vi "Global Log Event Example.vi"() -> ()   [LabVIEW 2017]
uses:
  user.lib/_NEVSTOP/Communicable State Machine(CSM)/_Support/Typedef/_CSM_GlobalLog_MSG.ctl
  user.lib/_NEVSTOP/Communicable State Machine(CSM)/_Support/Typedef/_CSM_Response Source Message.ctl
  user.lib/_NEVSTOP/Communicable State Machine(CSM)/_Support/Typedef/_CSM_GlobalLog_MSG_TYPE.ctl
  user.lib/_NEVSTOP/Communicable State Machine(CSM)/AdvanceAPI/CSM - Convert Error to Argument.vi
  user.lib/_NEVSTOP/Communicable State Machine(CSM)/_Support/GlobalEvent/GEvt-Generate with Rule Check.vi
  user.lib/_NEVSTOP/Communicable State Machine(CSM)/_Support/GlobalEvent/Cache-GEvt Refs.vi
  user.lib/_NEVSTOP/Communicable State Machine(CSM)/_Support/Common/Format Timestamp.vi
  user.lib/_NEVSTOP/Communicable State Machine(CSM)/AdvanceAPI/CSM - Make String Arguments Safe.vi
  user.lib/_NEVSTOP/Communicable State Machine(CSM)/_Support/ChangeFlag/FlagInstance-GEvt Refs.vi
  user.lib/_NEVSTOP/Communicable State Machine(CSM)/AdvanceAPI/CSM - Keywords.vi
  user.lib/_NEVSTOP/Communicable State Machine(CSM)/_Support/ChangeFlag/ChangeFlag-Read.vi
  user.lib/_NEVSTOP/Communicable State Machine(CSM)/_Support/GlobalEvent/LogFilter/LogFilter - Check.vi
  user.lib/_NEVSTOP/Communicable State Machine(CSM)/_Support/GlobalEvent/GEvt-Valid Subscribers.vi
  user.lib/_NEVSTOP/Communicable State Machine(CSM)/_Support/GlobalEvent/FGV-GlobalEventQueues(lvlibp).vi
  user.lib/_NEVSTOP/Communicable State Machine(CSM)/_Support/GlobalEvent/FGV-GlobalEventRef(lvlibp).vi
  user.lib/_NEVSTOP/Communicable State Machine(CSM)/_Support/ChangeFlag/ChangeFlagDB.vi
  user.lib/_NEVSTOP/Communicable State Machine(CSM)/_Support/GlobalEvent/LogFilter/LogFilter.lvclass
  user.lib/_NEVSTOP/Communicable State Machine(CSM)/Communicable State Machine.lvlib
panel:
  in  "Generate user log 3":bool
  in  "Generate user log 2":bool
  in  "Generate user log":bool
  in  "Generate an Error 2":bool
  in  "Generate an Error":bool
  out "State History":string
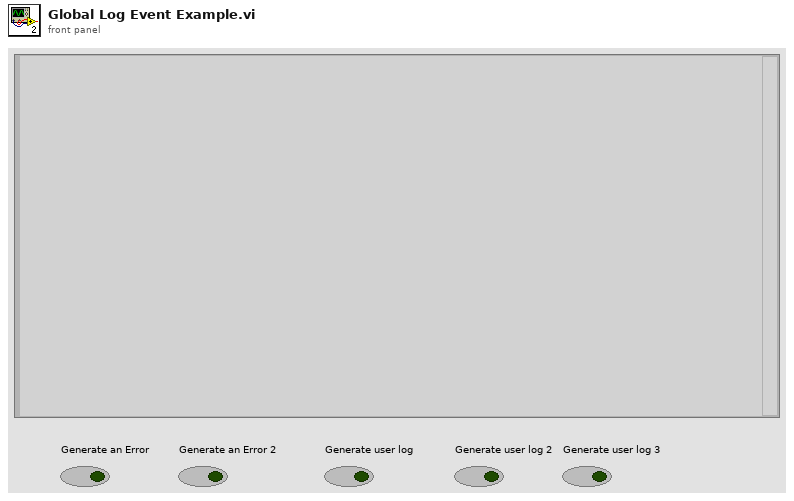
[diagram p1: front panel]
types:
  T1 = typedef "Communicable State Machine.lvlib/_CSM_GlobalLog_MSG.ctl" = cluster{"Name (\"\" to Use UUID)":string, "Current State":string, "Arguments":string, "Source Message":T2, "Source Module":string, "Complete(T)/Start(F)":bool, "LogType":T3, "Time Stamp":timestamp}
  T2 = typedef "Communicable State Machine.lvlib/_CSM_Response Source Message.ctl" = cluster{"‘State":string, "’Arguments":string, "’Error":errorcluster}
  T3 = typedef "Communicable State Machine.lvlib/_CSM_GlobalLog_MSG_TYPE.ctl" = enum16{"User Log", "State Change", "Status", "Interrupt", "Register", "Unregister", "Error Log", "Module Created", "Module Destroyed", "Async Message", "No-Rep Async Message", "Sync Message"}
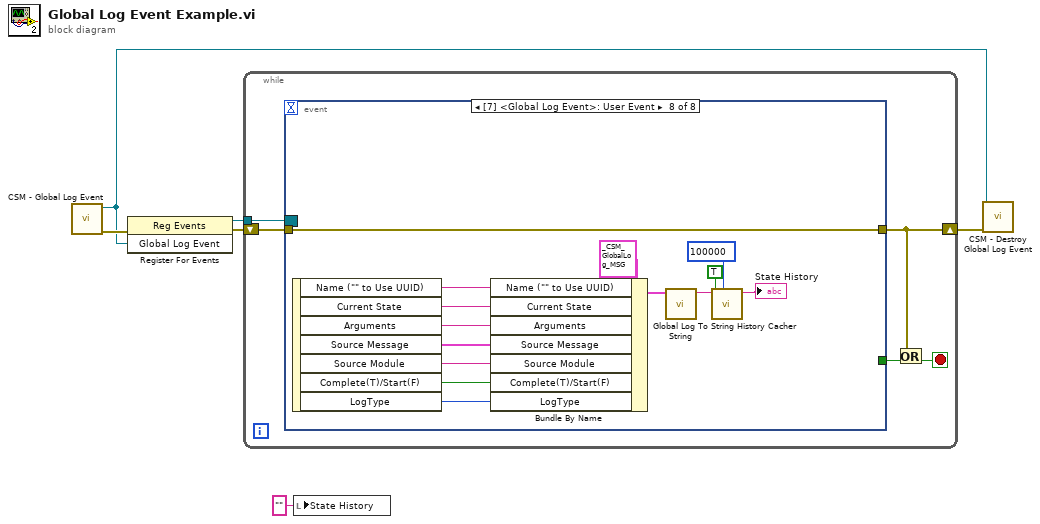
[diagram p0: block diagram]
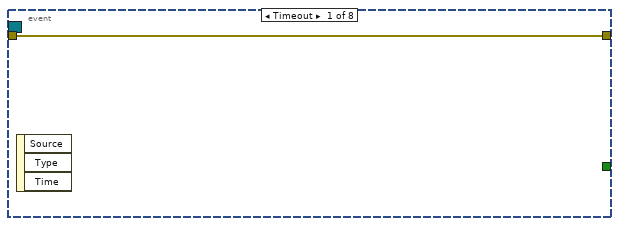
[diagram p2: hidden frame]
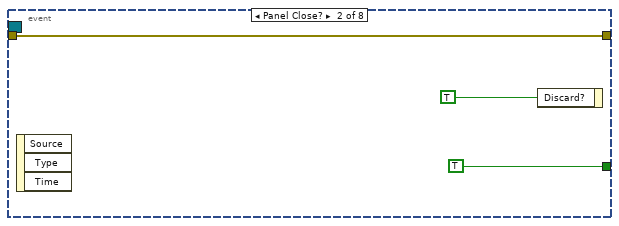
[diagram p3: hidden frame]
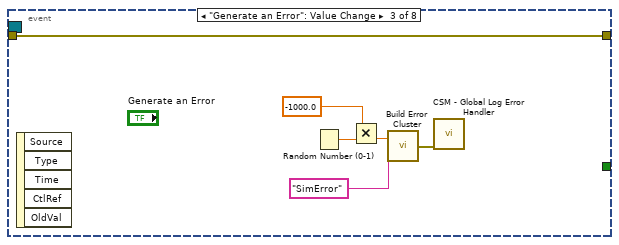
[diagram p4: hidden frame]
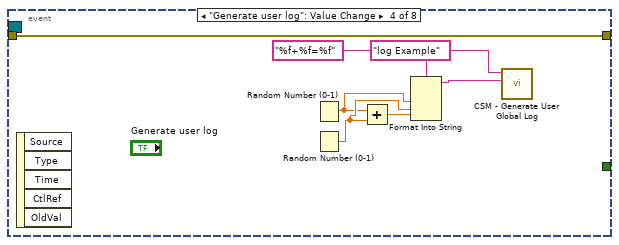
[diagram p5: hidden frame]
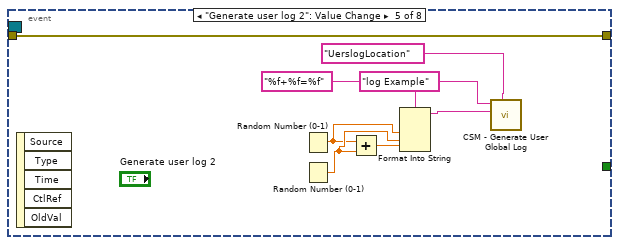
[diagram p6: hidden frame]
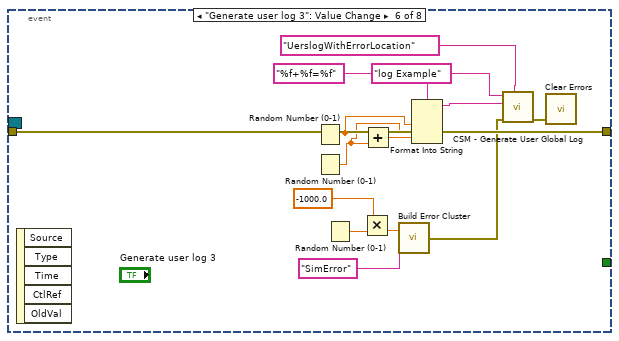
[diagram p7: hidden frame]
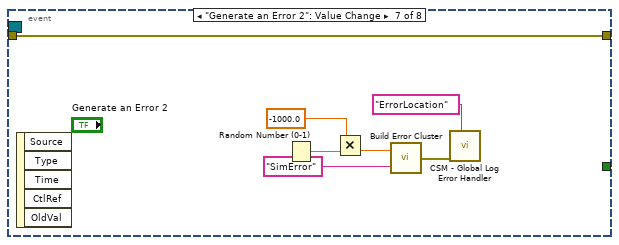
[diagram p8: hidden frame]
diagram:
  n1 = call "CSM - Global Log Event.vi"() -> ("error out"=w3:errorcluster, "Global Log Event"=w2:refnum<user-event>)  [unwired: 10 in]
  n2 = register-events(error in=w3, w2) -> (reference out=w6:refnum<event-registration>, error out=w5:errorcluster)  [unwired: 1 in]
  n3 = while {
    tunnel: w6 -> [w11]
    shift-right: [w8] -> w4
    shift-left: w5 -> [w10]
    stop <- w9 stop-if-true
    n4 = event shown="[7] <Global Log Event>: User Event" {
      selector: w11 -> [_ _ _ _ _ _ _ _]
      dyn-events: _ -> [_ _ _ _ _ _ _ _]
      timeout: _ -> [_ _ _ _ _ _ _ _]
      tunnel: w10 -> [w12 w15 w21 w28 w36 w50 w57 w71]
      tunnel: [w12 w15 w21 w28 w36 w50 w57 w71] -> w8
      tunnel: [_ TRUE ("Discard?") _ _ _ _ _ _] -> w7
      event Timeout {
        n5 = event-data() -> ()  [unwired: 1 in, 3 out]
      }
      event Panel Close? {
        n6 = event-data() -> ()  [unwired: 1 in, 3 out]
        n7 = event-data("Discard?"=TRUE) -> ()  [unwired: 1 in, 1 out]
      }
      event "Generate an Error": Value Change {
        n8 = event-data() -> ()  [unwired: 1 in, 5 out]
        n9 = Random Number (0-1)() -> (number: 0 to 1=w20:dbl)
        n10 = Multiply(x=-1000.0, y=w20) -> (x*y=w19:dbl)
        n11 = call "Build Error Cluster.vi"("String to Prepend to Source (\"\")"="SimError" ("String to Prepend to source (\"\")"), "Code"=w19) -> ("error out"=w16:errorcluster)
        n12 = call "CSM - Global Log Error Handler.vi"("Error In"=w16) -> ()  [unwired: 10 in, 1 out]
      }
      event "Generate user log": Value Change {
        n13 = event-data() -> ()  [unwired: 1 in, 5 out]
        n14 = Random Number (0-1)() -> (number: 0 to 1=w25:dbl)
        n15 = Random Number (0-1)() -> (number: 0 to 1=w26:dbl)
        n16 = Add(x=w25, y=w26) -> (x+y=w27:dbl)
        n17 = Format Into String(format string="%f+%f=%f", w25, w26, w27) -> (resulting string=w23:string)  [unwired: 2 in, 1 out]
        n18 = call "CSM - Generate User Global Log.vi"("Arguments"=w23, "Log"="log Example") -> ()  [unwired: 9 in, 1 out]
      }
      event "Generate user log 2": Value Change {
        n19 = event-data() -> ()  [unwired: 1 in, 5 out]
        n20 = Random Number (0-1)() -> (number: 0 to 1=w33:dbl)
        n21 = Random Number (0-1)() -> (number: 0 to 1=w34:dbl)
        n22 = Add(x=w33, y=w34) -> (x+y=w35:dbl)
        n23 = Format Into String(format string="%f+%f=%f", w33, w34, w35) -> (resulting string=w31:string)  [unwired: 2 in, 1 out]
        n24 = call "CSM - Generate User Global Log.vi"("Place (\"\" to Use VI's Name)"="UerslogLocation" ("Place(\"\" to use VI's Name)"), "Arguments"=w31, "Log"="log Example") -> ()  [unwired: 8 in, 1 out]
      }
      event "Generate user log 3": Value Change {
        n25 = event-data() -> ()  [unwired: 1 in, 5 out]
        n26 = Random Number (0-1)() -> (number: 0 to 1=w47:dbl)
        n27 = Random Number (0-1)() -> (number: 0 to 1=w48:dbl)
        n28 = Random Number (0-1)() -> (number: 0 to 1=w42:dbl)
        n29 = Multiply(x=-1000.0, y=w42) -> (x*y=w41:dbl)
        n30 = Add(x=w47, y=w48) -> (x+y=w49:dbl)
        n31 = call "Build Error Cluster.vi"("String to Prepend to Source (\"\")"="SimError" ("String to Prepend to source (\"\")"), "Code"=w41) -> ("error out"=w38:errorcluster)
        n32 = Format Into String(format string="%f+%f=%f", w47, w48, w49) -> (resulting string=w45:string)  [unwired: 2 in, 1 out]
        n33 = call "CSM - Generate User Global Log.vi"("Place (\"\" to Use VI's Name)"="UerslogWithErrorLocation" ("Place(\"\" to use VI's Name)"), "Error In"=w38, "Arguments"=w45, "Log"="log Example") -> ("error out"=w37:errorcluster)  [unwired: 7 in]
        n34 = call <vilib>:"Clear Errors.vi"("error in (no error)"=w37) -> ()  [unwired: 5 in, 2 out]
      }
      event "Generate an Error 2": Value Change {
        n35 = event-data() -> ()  [unwired: 1 in, 5 out]
        n36 = Random Number (0-1)() -> (number: 0 to 1=w56:dbl)
        n37 = Multiply(x=-1000.0, y=w56) -> (x*y=w55:dbl)
        n38 = call "Build Error Cluster.vi"("String to Prepend to Source (\"\")"="SimError" ("String to Prepend to source (\"\")"), "Code"=w55) -> ("error out"=w52:errorcluster)
        n39 = call "CSM - Global Log Error Handler.vi"("Place (\"\" to Use VI's Name)"="ErrorLocation" ("Place(\"\" to use VI's Name)"), "Error In"=w52) -> ()  [unwired: 9 in, 1 out]
      }
      event User Event {
        n40 = event-data() -> ("Name (\"\" to Use UUID)"=w66:string, "Current State"=w65:string, "Arguments"=w64:string, "Source Message"=w63:T2, "Source Module"=w62:string, "Complete(T)/Start(F)"=w61:bool, "LogType"=w60:T3)  [unwired: 1 in]
        n41 = Bundle By Name(cluster=T1 {"Name (\"\" to Use UUID)"="", "Current State"="", "Arguments"="", "Source Message"={"‘State"="", "’Arguments"="", "’Error"={"status"=FALSE, "code"=0, "source"=""}}, "Source Module"="", "Complete(T)/Start(F)"=FALSE, "LogType"=enum."State Change", "Time Stamp"=timestamp(0 s since 1904-01-01)} ("Cross CSM Data"), "Name (\"\" to Use UUID)"=w66, "Current State"=w65, "Arguments"=w64, "Source Message"=w63, "Source Module"=w62, "Complete(T)/Start(F)"=w61, "LogType"=w60) -> (w58:T1)
        n42 = call "Global Log To String.vi"("Log"=w58) -> ("Log String"=w67:string)  [unwired: 9 in]
        n43 = call "String History Cacher.vi"("Length"=100000 ("length"), "Include Timestamp? (T)"=TRUE ("Include Timestamp(F)"), "String"=w67) -> ("String Cache"=→"State History":string)  [unwired: 8 in]
      }
    }
    n44 = Or(x=w8, y=w7) -> (x .or. y?=w9:bool)
  }
  n45 = local write "State History"("" ("State History")) -> ()
  n46 = call "CSM - Destroy Global Log Event.vi"("Error In"=w4, "CSM Global Log Event"=w2) -> ()  [unwired: 9 in, 1 out]
